vi "conv_v_to_torr.vi"(11 "Scalar":dbl) -> (3 "Numeric":dbl)   [LabVIEW 2016]
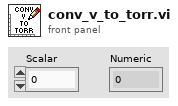
[diagram p1: front panel]
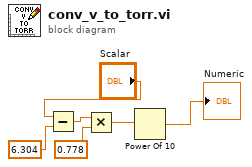
[diagram p0: block diagram]
diagram:
  n1 = Subtract(x="Scalar", y=6.304) -> (x-y=w2:dbl)
  n2 = Multiply(x=w2, y=0.778) -> (x*y=w4:dbl)
  n3 = Power Of 10(x=w4) -> (10^x=→"Numeric":dbl)
